vi "Method.vi"(4 "Input B":refnum<class "Abs_Numeric.lvclass">, 5 "Input A":refnum<class "Abs_I32 Integer.lvclass">) -> (1 "Result":T1)   [LabVIEW 2021, in "Subtract_I32.lvclass"]
uses:
  Subtract_I32.lvclass
  Abs_Types/I32 Integer/Abs_I32 Integer.lvclass
  Abs Type.ctl
  Abs_Types/Numeric/Abs_Numeric.lvclass
  C:/TSA/LV_Abstract/Source/Functions/Support/Function/Two Terminal/I32/AbsFunc_Two Term_I32.lvclass
  C:/Program Files (x86)/National Instruments/LabVIEW 2021/vi.lib/TSA/Abstract Data Classes/Abs_Types/I32 Integer/Abs_I32 Integer.lvclass
  Support/Function/Two Terminal/I32/AbsFunc_Two Term_I32.lvclass/AbsFunc_Two Term_I32.ctl
  Support/Function/Two Terminal/I32/Properties/Write Numeric A.vi
  Support/Function/Two Terminal/I32/Properties/Write Numeric B.vi
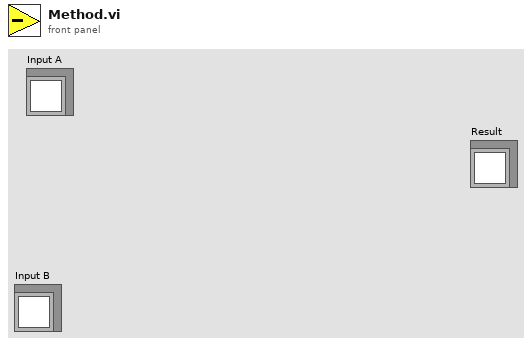
[diagram p1: front panel]
types:
  T1 = typedef "Subtract_I32.lvclass/Abs Type.ctl" = refnum<class "Abs_I32 Integer.lvclass">
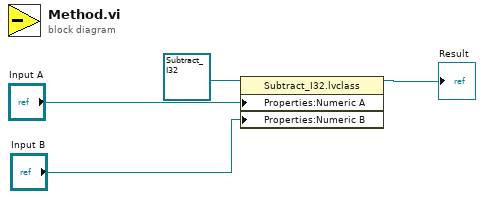
[diagram p0: block diagram]
diagram:
  n1 = property class="Subtract_I32.lvclass"(reference=refnum<class "Subtract_I32.lvclass"> refnum ("Subtract_DBL.lvclass"), "Properties:Numeric A"="Input A", "Properties:Numeric B"="Input B") -> (reference out=→"Result":refnum<class "Subtract_I32.lvclass">)  [unwired: 1 in, 1 out]
